vi "LSMcontroller_v56_from here for labview64bit.vi"() -> ()   [LabVIEW 2015] (continued)
                n2595 = call-poly <vilib>:"DAQmx Write.vi"("task/channels in"=w5605, "data"=w5596, "error in"=w5604) -> ("task out"=w5606:refnum<k21>, "error out"=w5607:errorcluster)  [unwired: 10 in, 1 out]
                n2596 = call <vilib>:"DAQmx Start Task.vi"("task/channels in"=w5606, "error in"=w5607) -> ("task out"=w5608:refnum<k21>, "error out"=w5609:errorcluster)  [unwired: 12 in]
                n2597 = call <vilib>:"DAQmx Stop Task.vi"("task/channels in"=w5608, "error in"=w5609) -> ("task out"=w5610:refnum<k21>, "error out"=w5611:errorcluster)  [unwired: 12 in]
                n2598 = call <vilib>:"DAQmx Clear Task.vi"("task in"=w5610, "error in"=w5611) -> ()  [unwired: 13 in, 1 out]
              }
            }
          }
          event "sealtest": Value Change {
            n2599 = event-data() -> ()  [unwired: 1 in, 6 out]
            n2600 = case shown="True" "sealtest" {
              frame False {
              }
              frame True {
                n2601 = stacked-sequence {
                  seq-local: [w5613 _ _ _ _ _] -> [_ w5646 _ w5698 _ _]
                  frame #0 {
                    n2602 = stacked-sequence {
                      tunnel: [_ w5625 _] -> w5613
                      frame #0 {
                        n2603 = call "2pparameters.vi"("command"="get") -> ("params out"=w5618:T12)  [unwired: 1 in]
                        n2604 = Unbundle By Name(w5618) -> ("autoshutter"=w5619:bool)
                        n2605 = local read "OCchecked?"() -> (w5616:bool)
                        n2606 = call "sealtestwfparams.vi"("command"="set") -> ()  [unwired: 6 in, 1 out]
                        n2607 = case shown="False" w5616 {
                          frame False {
                            n2608 = One Button Dialog(message="Is the OC gain correct?", button name ("OK")="ok") -> (true=w5620:bool)
                            n2609 = local write "OCchecked?"(w5620) -> ()
                          }
                          frame True {
                          }
                        }
                        n2610 = case shown="True" w5619 {
                          frame False {
                          }
                          frame True {
                            n2611 = call "shuttercontrol.vi"("command"="close") -> ()  [unwired: 1 in, 1 out]
                          }
                        }
                        n2612 = call "allAI-temp.vi"("command"=enum16{"get", "set", "clear", "append"}."clear") -> ()  [unwired: 3 in, 2 out]
                      }
                      frame #1 {
                        n2613 = call "sealtestwfparams.vi"("command"="get") -> ("Params out"=w5631:T25)  [unwired: 6 in]
                        n2614 = Unbundle By Name(w5631) -> ("AO parameters"=w5629:T1)
                        "AO parameters 2" <- w5629
                        n2615 = Index Array(array=w5629, index=0) -> (element=w5628:T26)
                        n2616 = call "generateRampedSquareWave_fromAOparameters.vi"("AO params"=w5628) -> ("Waveform"=w5624:waveform(dbl), "wflength"=w5625:i32)
                        "Waveform Graph" <- w5624
                        "wflength" <- w5625
                        n2617 = Build Array(w5624) -> (w5627:waveform(dbl)[])
                        n2618 = call "waveformssealtestbuffer.vi"("AO wf in"=w5627, "command"="set") -> ()  [unwired: 1 out]
                      }
                      frame #2 {
                        n2619 = local read "Vholding (mV)"() -> (w5634:sgl)
                        n2620 = local read "Current Clamp"() -> (w5640:bool)
                        n2621 = local read "Voltage Clamp"() -> (w5639:bool)
                        n2622 = local read "OCgain"() -> (w5635:sgl)
                        n2623 = local read "CC_ICgain"() -> (w5638:dbl)
                        n2624 = local read "holdon"() -> (w5633:bool)
                        n2625 = call "patchparameters.vi"("command"="get") -> ("Params out"=w5642:T15)  [unwired: 1 in]
                        n2626 = Bundle By Name(cluster=w5642, "VC"=w5639, "CC"=w5640, "CC_icg (pA/mv)"=w5638, "VC_icg (mV/mV)"=10.0, "OCG (mV/pA)"=w5635, "OVG (mV/mV)"=0.1, "Vhold (mV)"=w5634, "holdon"=w5633) -> (w5641:T15)
                        n2627 = call "patchparameters.vi"("Params in"=w5641, "command"="set") -> ()  [unwired: 1 out]
                      }
                    }
                  }
                  frame #1 {
                    w5645 = 2
                    n2628 = call "patchparameters.vi"("command"="get") -> ("Params out"=w5653:T15)  [unwired: 1 in]
                    n2629 = Unbundle By Name(w5653) -> ("holdon"=w5652:bool, "Vhold (mV)"=w5651:sgl, "CC_icg (pA/mv)"=w5659:sgl, "CC"=w5657:bool, "VC_icg (mV/mV)"=w5658:sgl)
                    n2630 = Select(t=w5659, s=w5657, f=w5658) -> (s? t:f=w5660:sgl)
                    n2631 = To Single Precision Float(number=0.001 ("y")) -> (single precision float=w5661:sgl)
                    n2632 = Compound Arithmetic op=MULTIPLY(w5651, w5660, w5661) -> (w5655:sgl)
                    n2633 = case shown="False" w5652 {
                      tunnel: w5655 -> [_ w5673]
                      tunnel: [0.0 w5673] -> w5648
                      frame False {
                      }
                      frame True {
                      }
                    }
                    n2634 = Greater Than 0?(x=w5645) -> (x > 0?=w5647:bool)
                    n2635 = case shown="True" w5647 {
                      tunnel: w5646 -> [_ w5662]
                      tunnel: w5645 -> [_ w5665]
                      frame False {
                      }
                      frame True {
                        n2636 = Initialize Array(sgl 0.0 ("element"), w5665, w5662) -> (w5663:sgl[][])
                        n2637 = call "allAI-temp.vi"("array in"=w5663, "command"=enum16{"get", "set", "clear", "append"}."set") -> ()  [unwired: 2 in, 2 out]
                      }
                    }
                    n2638 = flat-sequence {
                      tunnel: w5646 -> [w5669]
                      tunnel: w5646 -> [w5668]
                      tunnel: [w5668] -> w5650
                      tunnel: [w5667] -> w5649
                      tunnel: w5648 -> [w5667]
                      tunnel: w5650 -> [w5671]
                      tunnel: w5649 -> [w5670]
                      frame #0 {
                        n2639 = call "prepAI_sealtest.vi"("samples per channel"=w5669) -> ()  [unwired: 2 in]
                      }
                      frame #1 {
                        n2640 = call "prepAO_sealtest.vi"("Vhold"=w5670, "samples per channel"=w5671) -> ()  [unwired: 1 in]
                      }
                    }
                  }
                  frame #2 {
                    n2641 = stacked-sequence {
                      frame #0 {
                        n2642 = call "tempconfigAO.vi"("command"="get") -> ("Temp Config out"=w5677:T27)  [unwired: 1 in]
                        n2643 = Unbundle By Name(w5677) -> ("AO"=w5678:refnum<k21>[], "E_AO"=w5679:errorcluster[])
                        n2644 = for {
                          tunnel: w5678 -> [w5687] mode=indexing
                          tunnel: w5679 -> [w5686] mode=indexing
                          tunnel: [w5685] -> w5681 mode=indexing
                          tunnel: [w5684] -> w5682 mode=indexing
                          n2645 = call <vilib>:"DAQmx Start Task.vi"("task/channels in"=w5687, "error in"=w5686) -> ("task out"=w5685:refnum<k21>, "error out"=w5684:errorcluster)  [unwired: 12 in]
                        }
                        n2646 = call "tempconfigAO.vi"("command"="get") -> ("Temp Config out"=w5680:T27)  [unwired: 1 in]
                        n2647 = Bundle By Name(cluster=w5680, "AO"=w5681, "E_AO"=w5682) -> (w5683:T27)
                        n2648 = call "tempconfigAO.vi"("Temp Config in"=w5683, "command"="set") -> ()  [unwired: 1 out]
                      }
                      frame #1 {
                        n2649 = call "tempconfigAI.vi"("command"="get") -> ("Temp Config out"=w5689:T28)  [unwired: 1 in]
                        n2650 = Unbundle By Name(w5689) -> ("AI"=w5694:refnum<k21>, "E_AI"=w5695:errorcluster)
                        n2651 = call <vilib>:"DAQmx Start Task.vi"("task/channels in"=w5694, "error in"=w5695) -> ("task out"=w5696:refnum<k21>, "error out"=w5697:errorcluster)  [unwired: 12 in]
                        n2652 = call "tempconfigAI.vi"("command"="get") -> ("Temp Config out"=w5691:T28)  [unwired: 1 in]
                        n2653 = Bundle By Name(cluster=w5691, "AI"=w5696, "E_AI"=w5697) -> (w5693:T28)
                        n2654 = call "tempconfigAI.vi"("Temp Config in"=w5693, "command"="set") -> ()  [unwired: 1 out]
                      }
                    }
                  }
                  frame #3 {
                    n2655 = while {
                      tunnel: w5698 -> [w5699]
                      stop <- w5700 stop-if-true
                      n2656 = local read "sealtest"() -> (w5703:bool)
                      n2657 = Not(x=w5703) -> (.not. x?=w5702:bool)
                      n2658 = case shown="False" w5702 {
                        tunnel: w5699 -> [w5704 _]
                        frame False {
                          n2659 = stacked-sequence {
                            seq-local: [_ _ _ w5743 _ _] -> [_ _ _ _ w5799 _]
                            seq-local: [w5705 _ _ _ _ _] -> [_ w5714 _ w5736 w5784 w5819]
                            tunnel: w5704 -> [_ _ w5722 _ w5783 _]
                            frame #0 {
                              n2660 = call "patchparameters.vi"("command"="get") -> ("Params out"=w5712:T15)  [unwired: 1 in]
                              n2661 = local read "Vholding (mV)"() -> (w5709:sgl)
                              n2662 = Unbundle By Name(w5712) -> ("Vhold (mV)"=w5708:sgl, "holdon"=w5711:bool)
                              n2663 = local read "holdon"() -> (w5710:bool)
                              n2664 = Not Equal?(x=w5709, y=w5708) -> (x != y?=w5707:bool)
                              n2665 = Not Equal?(x=w5711, y=w5710) -> (x != y?=w5706:bool)
                              n2666 = Or(x=w5707, y=w5706) -> (x .or. y?=w5705:bool)
                            }
                            frame #1 {
                              n2667 = case shown="True" w5714 {
                                frame False {
                                }
                                frame True {
                                n2668 = local read "Vholding (mV)"() -> (w5717:sgl)
                                n2669 = local read "holdon"() -> (w5715:bool)
                                n2670 = call "patchparameters.vi"("command"="get") -> ("Params out"=w5718:T15)  [unwired: 1 in]
                                n2671 = Bundle By Name(cluster=w5718, "Vhold (mV)"=w5717, "holdon"=w5715) -> (w5716:T15)
                                n2672 = call "patchparameters.vi"("Params in"=w5716, "command"="set") -> ()  [unwired: 1 out]
                                }
                              }
                            }
                            frame #2 {
                              n2673 = call "tempconfigAI.vi"("command"="get") -> ("Temp Config out"=w5732:T28)  [unwired: 1 in]
                              n2674 = Unbundle By Name(w5732) -> ("AI"=w5731:refnum<k21>, "E_AI"=w5730:errorcluster)
                              n2675 = call-poly <vilib>:"DAQmx Read.vi"("task/channels in"=w5731, "number of samples per channel"=w5722, "timeout"=10.0, "error in"=w5730) -> ("task out"=w5726:refnum<k21>, "data"=w5723:i16[][], "error out"=w5735:errorcluster)  [unwired: 9 in]
                              n2676 = call "tempconfigAI.vi"("command"="get") -> ("Temp Config out"=w5727:T28)  [unwired: 1 in]
                              n2677 = Bundle By Name(cluster=w5727, "AI"=w5726, "E_AI"=w5735) -> (w5734:T28)
                              n2678 = To Single Precision Float(number=w5723) -> (single precision float=w5725:sgl[][])
                              n2679 = call "tempconfigAI.vi"("Temp Config in"=w5734, "command"="set") -> ()  [unwired: 1 out]
                              n2680 = call "allAI-temp.vi"("array in"=w5725, "command"=enum16{"get", "set", "clear", "append"}."set") -> ()  [unwired: 2 in, 2 out]
                            }
                            frame #3 {
                              n2681 = case shown="True" w5736 {
                                frame False {
                                }
                                frame True {
                                n2682 = call "tempconfigAO.vi"("command"="get") -> ("Temp Config out"=w5776:T27)  [unwired: 1 in]
                                n2683 = Unbundle By Name(w5776) -> ("AO"=w5775:refnum<k21>[], "E_AO"=w5774:errorcluster[])
                                n2684 = call "tempconfigAI.vi"("command"="get") -> ("Temp Config out"=w5763:T28)  [unwired: 1 in]
                                n2685 = Unbundle By Name(w5763) -> ("AI"=w5764:refnum<k21>, "E_AI"=w5765:errorcluster)
                                n2686 = for {
                                tunnel: w5775 -> [w5780] mode=indexing
                                tunnel: w5774 -> [w5779] mode=indexing
                                tunnel: [w5778] -> w5770 mode=indexing
                                n2687 = call <vilib>:"DAQmx Stop Task.vi"("task/channels in"=w5780, "error in"=w5779) -> ("task out"=w5781:refnum<k21>, "error out"=w5782:errorcluster)  [unwired: 12 in]
                                n2688 = call <vilib>:"DAQmx Clear Task.vi"("task in"=w5781, "error in"=w5782) -> ("error out"=w5778:errorcluster)  [unwired: 13 in]
                                }
                                n2689 = call <vilib>:"DAQmx Stop Task.vi"("task/channels in"=w5764, "error in"=w5765) -> ("task out"=w5761:refnum<k21>, "error out"=w5760:errorcluster)  [unwired: 12 in]
                                n2690 = call <vilib>:"DAQmx Clear Task.vi"("task in"=w5761, "error in"=w5760) -> ("error out"=w5759:errorcluster)  [unwired: 13 in]
                                n2691 = call "tempconfigAO.vi"("command"="get") -> ("Temp Config out"=w5771:T27)  [unwired: 1 in]
                                n2692 = Bundle By Name(cluster=w5771, "E_AO"=w5770) -> (w5769:T27)
                                n2693 = call "tempconfigAI.vi"("command"="get") -> ("Temp Config out"=w5767:T28)  [unwired: 1 in]
                                n2694 = Bundle By Name(cluster=w5767, "E_AI"=w5759) -> (w5758:T28)
                                n2695 = call "tempconfigAO.vi"("Temp Config in"=w5769, "command"="set") -> ()  [unwired: 1 out]
                                n2696 = call "tempconfigAI.vi"("Temp Config in"=w5758, "command"="set") -> ()  [unwired: 1 out]
                                }
                              }
                              n2697 = call "allAI-temp.vi"("command"=enum16{"get", "set", "clear", "append"}."get") -> ("array out"=w5740:sgl[][])  [unwired: 3 in, 1 out]
                              n2698 = call "tempconfigAI.vi"("command"="get") -> ("Temp Config out"=w5753:T28)  [unwired: 1 in]
                              n2699 = call "tempconfigAI.vi"("command"="get") -> ("Temp Config out"=w5755:T28)  [unwired: 1 in]
                              n2700 = Unbundle By Name(w5753) -> ("header"=w5751:dbl[])
                              n2701 = Unbundle By Name(w5755) -> ("header"=w5757:dbl[])
                              n2702 = Index Array(array=w5740, index (row) #1=0 ("index (row)"), index (row) #2=1 ("index (row)")) -> (element #1=w5738:sgl[], element #2=w5737:sgl[])  [unwired: 2 in]
                              n2703 = local read "OCgain"() -> (w5745:sgl)
                              n2704 = call "Unscaledtoscaled.vi"("Unscaled Data"=w5738, "Header Information"=w5751) -> ("Array"=w5750:sgl[])  [unwired: 1 in]
                              n2705 = call "Unscaledtoscaled.vi"("Unscaled Data"=w5737, "Header Information"=w5757) -> ("Array"=w5754:sgl[])  [unwired: 1 in]
                              n2706 = Multiply(x=w5750, y=0.1) -> (x*y=w5747:dbl[])
                              n2707 = Divide(x=w5754, y=w5745) -> (x/y=w5746:sgl[])
                              n2708 = Build Array(w5747, w5746) -> (w5749:dbl[][])
                              n2709 = Multiply(x=w5749, y=1000.0) -> (x*y=w5743:dbl[][])
                              "Patch readout" <- w5743
                            }
                            frame #4 {
                              n2710 = case shown="True" w5784 {
                                tunnel: w5783 -> [_ w5800]
                                frame False {
                                }
                                frame True {
                                n2711 = call "patchparameters.vi"("command"="get") -> ("Params out"=w5804:T15)  [unwired: 1 in]
                                n2712 = Unbundle By Name(w5804) -> ("holdon"=w5803:bool, "Vhold (mV)"=w5802:sgl, "CC_icg (pA/mv)"=w5810:sgl, "CC"=w5808:bool, "VC_icg (mV/mV)"=w5809:sgl)
                                n2713 = Select(t=w5810, s=w5808, f=w5809) -> (s? t:f=w5811:sgl)
                                n2714 = To Single Precision Float(number=0.001 ("y")) -> (single precision float=w5812:sgl)
                                n2715 = Compound Arithmetic op=MULTIPLY(w5802, w5811, w5812) -> (w5806:sgl)
                                n2716 = case shown="False" w5803 {
                                tunnel: w5806 -> [_ w5817]
                                tunnel: [0.0 w5817] -> w5801
                                frame False {
                                }
                                frame True {
                                }
                                }
                                n2717 = flat-sequence {
                                tunnel: w5800 -> [w5813]
                                tunnel: w5801 -> [w5815]
                                tunnel: w5800 -> [w5814]
                                frame #0 {
                                n2718 = call "prepAI_sealtest.vi"("samples per channel"=w5813) -> ()  [unwired: 2 in]
                                }
                                frame #1 {
                                n2719 = call "prepAO_sealtest.vi"("Vhold"=w5815, "samples per channel"=w5814) -> ()  [unwired: 1 in]
                                }
                                }
                                }
                              }
                              n2720 = call "sealtestwfparams.vi"("command"="get") -> ("Params out"=w5789:T25)  [unwired: 6 in]
                              n2721 = Unbundle By Name(w5789) -> ("AO parameters"=w5790:T1)
                              n2722 = Index Array(array=w5790, index=0) -> (element=w5792:T26)
                              n2723 = Unbundle By Name(w5792) -> ("Cycles"=w5787:dbl, "Start amplitude (V)"=w5786:dbl, "Sampling frequency (Hz)"=w5785:dbl)
                              n2724 = local read "fitpoints"() -> (w5794:dbl)
                              n2725 = script code="V=data(:,2);\nI=data(:,1);\ntres=mean(V);\nspc=(nsamp./ncyc);\nV=V(spc+1:end-spc);\nI=I(spc+1:end-spc);\ndV=mean(V(V>tres))-mean(V(V<tres))\nIcyc=reshape(I,[spc ncyc-2]);\nIcyc=Icyc';\nIcyc=mean(Icyc,1);\ndIss=mean(Icyc(floor(spc*0.15):floor(spc/2)-2))-mean(Icyc(spc*0.65:spc-2))\nRm=dV*1e3/dIss;\n[maxi,ind]=max(Icyc);\nIfit=Icyc(ind+1:ind+1+points-1)-0.5*(mean(Icyc(floor(spc*0.15):floor(spc/2)-2))+mean(Icyc(spc*0.65:spc-2)))\nt=(3:points-1+3)./srate*1000;\nt=t';\nIfit=Ifit';\nc=fit(t,Ifit, 'exp1');\ncoeffs=coeffvalues(c);\nIa=coeffs(1);\nRa=dV*1e3./Ia/2;\ntau=-1./coeffs(2);\ncap=tau/Ra*1000;"("data"=w5799, "nsamp"=w5783, "ncyc"=w5787, "maxV"=w5786, "points"=w5794, "srate"=w5785) -> ("Icyc"=w5798:dbl[], "Rm"=w5796:dbl, "Ra"=w5795:dbl, "cap"=w5793:dbl)  [unwired: 1 in, 1 out]
                              n2726 = local read "set as Rp?"() -> (w5797:bool)
                              n2727 = local write "Rmembrane (MOhm)"(w5796) -> ()
                              n2728 = case shown="True" w5797 {
                                tunnel: w5796 -> [_ w5818]
                                frame False {
                                }
                                frame True {
                                n2729 = local write "Rpipette (MOhm)"(w5818) -> ()
                                }
                              }
                              n2730 = local write "Cmembrane"(w5793) -> ()
                              n2731 = local write "Racces (MOhm)"(w5795) -> ()
                              n2732 = local write "Ifit"(w5798) -> ()
                            }
                            frame #5 {
                              n2733 = local read "set as Rp?"() -> (w5820:bool)
                              n2734 = case shown="True" w5819 {
                                frame False {
                                }
                                frame True {
                                n2735 = call "tempconfigAO.vi"("command"="get") -> ("Temp Config out"=w5827:T27)  [unwired: 1 in]
                                n2736 = Unbundle By Name(w5827) -> ("AO"=w5826:refnum<k21>[], "E_AO"=w5825:errorcluster[])
                                n2737 = call "tempconfigAI.vi"("command"="get") -> ("Temp Config out"=w5832:T28)  [unwired: 1 in]
                                n2738 = Unbundle By Name(w5832) -> ("AI"=w5837:refnum<k21>, "E_AI"=w5838:errorcluster)
                                n2739 = for {
                                tunnel: w5826 -> [w5844] mode=indexing
                                tunnel: w5825 -> [w5843] mode=indexing
                                tunnel: [w5842] -> w5823 mode=indexing
                                tunnel: [w5841] -> w5822 mode=indexing
                                n2740 = call <vilib>:"DAQmx Start Task.vi"("task/channels in"=w5844, "error in"=w5843) -> ("task out"=w5842:refnum<k21>, "error out"=w5841:errorcluster)  [unwired: 12 in]
                                }
                                n2741 = call <vilib>:"DAQmx Start Task.vi"("task/channels in"=w5837, "error in"=w5838) -> ("task out"=w5839:refnum<k21>, "error out"=w5840:errorcluster)  [unwired: 12 in]
                                n2742 = call "tempconfigAO.vi"("command"="get") -> ("Temp Config out"=w5824:T27)  [unwired: 1 in]
                                n2743 = call "tempconfigAI.vi"("command"="get") -> ("Temp Config out"=w5834:T28)  [unwired: 1 in]
                                n2744 = Bundle By Name(cluster=w5824, "AO"=w5823, "E_AO"=w5822) -> (w5821:T27)
                                n2745 = Bundle By Name(cluster=w5834, "AI"=w5839, "E_AI"=w5840) -> (w5836:T28)
                                n2746 = call "tempconfigAI.vi"("Temp Config in"=w5836, "command"="set") -> ()  [unwired: 1 out]
                                n2747 = call "tempconfigAO.vi"("Temp Config in"=w5821, "command"="set") -> ()  [unwired: 1 out]
                                }
                              }
                              n2748 = case shown="True" w5820 {
                                frame False {
                                }
                                frame True {
                                n2749 = local write "set as Rp?"(FALSE ("set as Rp?")) -> ()
                                }
                              }
                            }
                          }
                        }
                        frame True {
                        }
                      }
                      n2750 = local read "sealtest"() -> (w5701:bool)
                      n2751 = Not(x=w5701) -> (.not. x?=w5700:bool)
                    }
                  }
                  frame #4 {
                    n2752 = call "tempconfigAO.vi"("command"="get") -> ("Temp Config out"=w5871:T27)  [unwired: 1 in]
                    n2753 = Unbundle By Name(w5871) -> ("AO"=w5870:refnum<k21>[], "E_AO"=w5869:errorcluster[])
                    n2754 = call "configuration.vi"("command"="get") -> ("config out"=w5852:T13)  [unwired: 2 in, 1 out]
                    n2755 = call "tempconfigAI.vi"("command"="get") -> ("Temp Config out"=w5858:T28)  [unwired: 1 in]
                    n2756 = Unbundle By Name(w5852) -> ("Device 1 sampleclock out"=w5849:tag, "Device 1 Starttrigger out"=w5848:tag)
                    n2757 = Unbundle By Name(w5858) -> ("AI"=w5859:refnum<k21>, "E_AI"=w5860:errorcluster)
                    n2758 = for {
                      tunnel: w5870 -> [w5875] mode=indexing
                      tunnel: w5869 -> [w5874] mode=indexing
                      tunnel: [w5873] -> w5865 mode=indexing
                      n2759 = call <vilib>:"DAQmx Stop Task.vi"("task/channels in"=w5875, "error in"=w5874) -> ("task out"=w5876:refnum<k21>, "error out"=w5877:errorcluster)  [unwired: 12 in]
                      n2760 = call <vilib>:"DAQmx Clear Task.vi"("task in"=w5876, "error in"=w5877) -> ("error out"=w5873:errorcluster)  [unwired: 13 in]
                    }
                    n2761 = call <vilib>:"DAQmx Stop Task.vi"("task/channels in"=w5859, "error in"=w5860) -> ("task out"=w5856:refnum<k21>, "error out"=w5855:errorcluster)  [unwired: 12 in]
                    n2762 = call <vilib>:"DAQmx Disconnect Terminals.vi"("source terminal"=tag "/Dev1/ai/SampleClock", "destination terminal"=w5849) -> ("error out"=w5846:errorcluster)  [unwired: 13 in]
                    n2763 = call <vilib>:"DAQmx Clear Task.vi"("task in"=w5856, "error in"=w5855) -> ("error out"=w5854:errorcluster)  [unwired: 13 in]
                    n2764 = call "tempconfigAO.vi"("command"="get") -> ("Temp Config out"=w5866:T27)  [unwired: 1 in]
                    n2765 = Bundle By Name(cluster=w5866, "E_AO"=w5865) -> (w5864:T27)
                    n2766 = call "tempconfigAI.vi"("command"="get") -> ("Temp Config out"=w5862:T28)  [unwired: 1 in]
                    n2767 = Bundle By Name(cluster=w5862, "E_AI"=w5854) -> (w5853:T28)
                    n2768 = call "tempconfigAO.vi"("Temp Config in"=w5864, "command"="set") -> ()  [unwired: 1 out]
                    n2769 = call <vilib>:"DAQmx Disconnect Terminals.vi"("source terminal"=tag "/Dev1/ai/StartTrigger", "destination terminal"=w5848, "error in"=w5846) -> ()  [unwired: 12 in, 1 out]
                    n2770 = call "tempconfigAI.vi"("Temp Config in"=w5853, "command"="set") -> ()  [unwired: 1 out]
                  }
                  frame #5 {
                    w5880 = T23 4 items=["no dialog", "OK message", "continue or stop message", "OK message + warnings", "continue/stop + warnings"] ("type of dialog (OK msg:1)")
                    n2771 = call "displayerrors.vi"() -> ("error IO"=w5879:errorcluster)
                    n2772 = call "zeropatch.vi"() -> ()  [unwired: 12 in]
                    n2773 = call <vilib>:"Simple Error Handler.vi"("type of dialog (OK msg:1)"=w5880, "error in (no error)"=w5879) -> ("error out"=w5878:errorcluster)  [unwired: 3 in, 4 out]
                    n2774 = call <vilib>:"Clear Errors.vi"("error in (no error)"=w5878) -> ()  [unwired: 5 in, 2 out]
                  }
                }
              }
            }
          }
          event "Current Clamp": Value Change {
            n2775 = event-data() -> ()  [unwired: 1 in, 6 out]
            n2776 = local read "Current Clamp"() -> (w5885:bool)
            n2777 = property on="Vholding (mV)" class="DigNum (strict)"("Caption.Text"="Ihold (pA)") -> ()  [unwired: 2 in, 2 out]
            n2778 = Not(x=w5885) -> (.not. x?=w5884:bool)
            n2779 = property on="Voltage Clamp" class="Bool (strict)"("Value"=w5884) -> ()  [unwired: 2 in, 2 out]
            n2780 = One Button Dialog(message="Have you switched the HEKA to CC and changed the external input cable?", button name ("OK")="Ok") -> ()  [unwired: 1 out]
          }
          event "Voltage Clamp": Value Change {
            n2781 = event-data() -> ()  [unwired: 1 in, 6 out]
            n2782 = local read "Voltage Clamp"() -> (w5890:bool)
            n2783 = Not(x=w5890) -> (.not. x?=w5889:bool)
            n2784 = property on="Current Clamp" class="Bool (strict)"("Value"=w5889) -> ()  [unwired: 2 in, 2 out]
            n2785 = One Button Dialog(message="Have you switched the HEKA to VC and changed the external input cable?", button name ("OK")="Ok") -> ()  [unwired: 1 out]
            n2786 = property on="Vholding (mV)" class="DigNum (strict)"("Caption.Text"="Vhold (mV)") -> ()  [unwired: 2 in, 2 out]
          }
          event "OCgain": Value Change {
            n2787 = event-data() -> ()  [unwired: 1 in, 6 out]
            n2788 = local read "OCgain"() -> (w5893:sgl)
            n2789 = Less?(x=w5893, y=0.3) -> (x < y?=w5891:bool)
            n2790 = case shown="True" w5891 {
              frame False {
                w5894 = 10.0 items=["0.1"=10.0, "10"=0.1] ("CC_ICgain")
                n2791 = local write "CC_ICgain"(w5894) -> ()
              }
              frame True {
                w5895 = 0.1 items=["0.1"=10.0, "10"=0.1] ("CC_ICgain")
                n2792 = local write "CC_ICgain"(w5895) -> ()
              }
            }
          }
          event "holdon": Value Change {
            n2793 = event-data() -> ()  [unwired: 1 in, 6 out]
            n2794 = stacked-sequence {
              frame #0 {
                n2795 = local read "Vholding (mV)"() -> (w5899:sgl)
                n2796 = local read "holdon"() -> (w5896:bool)
                n2797 = call "patchparameters.vi"("command"="get") -> ("Params out"=w5900:T15)  [unwired: 1 in]
                n2798 = Bundle By Name(cluster=w5900, "Vhold (mV)"=w5899, "holdon"=w5896) -> (w5897:T15)
                n2799 = call "patchparameters.vi"("Params in"=w5897, "command"="set") -> ()  [unwired: 1 out]
              }
              frame #1 {
                n2800 = call "zeropatch.vi"() -> ()  [unwired: 12 in]
              }
            }
          }
          event "Vholding (mV)": Value Change {
            n2801 = event-data() -> ()  [unwired: 1 in, 6 out]
            n2802 = local read "holdon"() -> (w5902:bool)
            n2803 = case shown="True" w5902 {
              frame False {
              }
              frame True {
                n2804 = stacked-sequence {
                  frame #0 {
                    n2805 = local read "Vholding (mV)"() -> (w5905:sgl)
                    n2806 = local read "holdon"() -> (w5906:bool)
                    n2807 = call "patchparameters.vi"("command"="get") -> ("Params out"=w5907:T15)  [unwired: 1 in]
                    n2808 = Bundle By Name(cluster=w5907, "Vhold (mV)"=w5905, "holdon"=w5906) -> (w5903:T15)
                    n2809 = call "patchparameters.vi"("Params in"=w5903, "command"="set") -> ()  [unwired: 1 out]
                  }
                  frame #1 {
                    n2810 = call "zeropatch.vi"() -> ()  [unwired: 12 in]
                  }
                }
              }
            }
          }
          event "readpatch": Value Change {
            n2811 = event-data() -> ("NewVal"=w5909:bool)  [unwired: 1 in, 5 out]
            n2812 = case shown="True" w5909 {
              frame False {
              }
              frame True {
                n2813 = stacked-sequence {
                  frame #0 {
                    n2814 = stacked-sequence {
                      frame #0 {
                        n2815 = call "2pparameters.vi"("command"="get") -> ("params out"=w5911:T12)  [unwired: 1 in]
                        n2816 = Unbundle By Name(w5911) -> ("autoshutter"=w5912:bool)
                        n2817 = case shown="True" w5912 {
                          frame False {
                          }
                          frame True {
                            n2818 = call "shuttercontrol.vi"("command"="close") -> ()  [unwired: 1 in, 1 out]
                          }
                        }
                      }
                      frame #1 {
                        n2819 = local read "Voltage Clamp"() -> (w5919:bool)
                        n2820 = local read "Current Clamp"() -> (w5920:bool)
                        n2821 = local read "Vholding (mV)"() -> (w5914:sgl)
                        n2822 = local read "CC_ICgain"() -> (w5918:dbl)
                        n2823 = local read "OCgain"() -> (w5915:sgl)
                        n2824 = call "patchparameters.vi"("command"="get") -> ("Params out"=w5922:T15)  [unwired: 1 in]
                        n2825 = Bundle By Name(cluster=w5922, "VC"=w5919, "CC"=w5920, "CC_icg (pA/mv)"=w5918, "VC_icg (mV/mV)"=10.0, "OCG (mV/pA)"=w5915, "OVG (mV/mV)"=0.1, "Vhold (mV)"=w5914) -> (w5921:T15)
                        n2826 = call "patchparameters.vi"("Params in"=w5921, "command"="set") -> ()  [unwired: 1 out]
                      }
                      frame #2 {
                        w5933 = 10123 items=["Finite Samples"=10178, "Continuous Samples"=10123, "Hardware Timed Single Point"=12522] ("sample mode")
                        n2827 = call "configuration.vi"("command"="get") -> ("config out"=w5928:T13)  [unwired: 2 in, 1 out]
                        n2828 = Unbundle By Name(w5928) -> ("Vp"=w5927:i32, "Ip"=w5926:i32)
                        n2829 = call "2pparameters.vi"("command"="get") -> ("params out"=w5936:T12)  [unwired: 1 in]
                        n2830 = Build Array(w5927, w5926) -> (w5925:i32[])
                        n2831 = Bundle By Name(cluster=w5936, "srate"=10000.0, "refreshbuffer"=500, "timeout"=10.0, "sample mode"=w5933, "aAI"=w5925) -> (w5934:T12)
                        n2832 = call "2pparameters.vi"("Params in"=w5934, "command"="set") -> ()  [unwired: 1 out]
                      }
                    }
                  }
                  frame #1 {
                    n2833 = while {
                      stop <- w5938 stop-if-true
                      n2834 = local read "readpatch"() -> (w5940:bool)
                      n2835 = case shown="True" w5940 {
                        frame False {
                        }
                        frame True {
                          n2836 = stacked-sequence {
                            frame #0 {
                              n2837 = local read "Vholding (mV)"() -> (w5943:sgl)
                              n2838 = local read "holdon"() -> (w5941:bool)
                              n2839 = call "patchparameters.vi"("command"="get") -> ("Params out"=w5944:T15)  [unwired: 1 in]
                              n2840 = Bundle By Name(cluster=w5944, "Vhold (mV)"=w5943, "holdon"=w5941) -> (w5942:T15)
                              n2841 = call "patchparameters.vi"("Params in"=w5942, "command"="set") -> ()  [unwired: 1 out]
                            }
                            frame #1 {
                              n2842 = call "zeropatch.vi"() -> ()  [unwired: 12 in]
                            }
                            frame #2 {
                              n2843 = call "prepAI_ttv2.vi"() -> ()  [unwired: 2 in, 1 out]
                            }
                            frame #3 {
                              n2844 = call "runAI_tt.vi"() -> ()  [unwired: 12 in]
                            }
                            frame #4 {
                              n2845 = call "collectAI_tt_V2.vi"() -> ()  [unwired: 4 in]
                            }
                            frame #5 {
                              n2846 = call "stoperaseAI_tt.vi"() -> ()  [unwired: 12 in]
                            }
                            frame #6 {
                              n2847 = call "tempconfigAI.vi"("command"="get") -> ("Temp Config out"=w5962:T28)  [unwired: 1 in]
                              n2848 = Unbundle By Name(w5962) -> ("header"=w5952:dbl[])
                              n2849 = call "allAI-temp.vi"("command"=enum16{"get", "set", "clear", "append"}."get") -> ("array out"=w5953:sgl[][])  [unwired: 3 in, 1 out]
                              n2850 = call "Unscaledtoscaled2D.vi"("Unscaled Data"=w5953, "Header Information"=w5952) -> ("Array"=w5951:sgl[][])  [unwired: 1 in]
                              n2851 = local read "OCgain"() -> (w5963:sgl)
                              n2852 = Index Array(array=w5951, index (row) #1=0 ("index (row)"), index (row) #2=1 ("index (row)")) -> (element #1=w5948:sgl[], element #2=w5947:sgl[])  [unwired: 2 in]
                              n2853 = Divide(x=w5948, y=w5963) -> (x/y=w5957:sgl[])
                              n2854 = Multiply(x=w5947, y=sgl 0.1) -> (x*y=w5956:sgl[])
                              n2855 = Build Array(w5957, w5956) -> (w5960:sgl[][])
                              n2856 = Multiply(x=w5960, y=sgl 1000.0) -> (x*y=w5955:sgl[][])
                              n2857 = local write "Patch readout"(w5955) -> ()
                            }
                          }
                        }
                      }
                      n2858 = local read "readpatch"() -> (w5939:bool)
                      n2859 = Not(x=w5939) -> (.not. x?=w5938:bool)
                    }
                  }
                  frame #2 {
                    w5966 = T23 4 items=["no dialog", "OK message", "continue or stop message", "OK message + warnings", "continue/stop + warnings"] ("type of dialog (OK msg:1)")
                    n2860 = call "displayerrors.vi"() -> ("error IO"=w5965:errorcluster)
                    n2861 = call <vilib>:"Simple Error Handler.vi"("type of dialog (OK msg:1)"=w5966, "error in (no error)"=w5965) -> ("error out"=w5964:errorcluster)  [unwired: 3 in, 4 out]
                    n2862 = call <vilib>:"Clear Errors.vi"("error in (no error)"=w5964) -> ()  [unwired: 5 in, 2 out]
                  }
                  frame #3 {
                    n2863 = call "zeropatch.vi"() -> ()  [unwired: 12 in]
                  }
                  frame #4 {
                    n2864 = disable-structure shown="Disabled" {
                      frame Disabled {
                        n2865 = local read item#-1() -> (w5972)
                        n2866 = local read item#-1() -> (w5971)
                        n2867 = local read item#-1() -> (w5968)
                        n2868 = local read item#-1() -> (w5970)
                        n2869 = local read item#-1() -> (w5969)
                        n2870 = local read item#-1() -> (w5967)
                        n2871 = call "waveformparamsv2.vi"("command"="get") -> ("Params out"=w5974:T24)  [unwired: 1 in]
                        n2872 = Bundle By Name(cluster=w5974, "patch"=w5972, "laserAO"=w5971, "shutter"=w5970, "488"=w5969, "532"=w5968, "640"=w5967) -> (w5973:T24)
                        n2873 = call "waveformparamsv2.vi"("Params in"=w5973, "command"="set") -> ()  [unwired: 1 out]
                      }
                      frame Enabled {
                      }
                    }
                  }
                  frame #5 {
                    n2874 = call "2pparameters.vi"("command"="get") -> ("params out"=w5978:T12)  [unwired: 1 in]
                    n2875 = Unbundle By Name(w5978) -> ("autoshutter"=w5979:bool)
                    n2876 = case shown="True" w5979 {
                      frame False {
                      }
                      frame True {
                        n2877 = call "shuttercontrol.vi"("command"="close") -> ()  [unwired: 1 in, 1 out]
                      }
                    }
                  }
                }
              }
            }
          }
          event "AI channels": Value Change {
            n2878 = event-data() -> ()  [unwired: 1 in, 6 out]
            n2879 = local read "CI channels"() -> (w5988:i32[])
            n2880 = local read "AI channels"() -> (w5989:i32[])
            n2881 = call "configuration.vi"("command"="get") -> ("config out"=w5982:T13)  [unwired: 2 in, 1 out]
            n2882 = Unbundle By Name(w5982) -> ("CI names"=w5983:string[], "AI names"=w5984:string[])
            n2883 = for {
              tunnel: w5988 -> [w5994] mode=indexing
              tunnel: w5983 -> [w5995]
              tunnel: [w5993] -> w5985 mode=indexing
              n2884 = Index Array(array=w5995, index=w5994) -> (element=w5993:string)
            }
            n2885 = for {
              tunnel: w5989 -> [w5991] mode=indexing
              tunnel: w5984 -> [w5992]
              tunnel: [w5990] -> w5986 mode=indexing
              n2886 = Index Array(array=w5992, index=w5991) -> (element=w5990:string)
            }
            n2887 = Build Array (concatenate)(w5985, w5986) -> (w5987:string[])
            n2888 = property on="image1list" class="Ring (strict)"("Strings []"=w5987) -> ()  [unwired: 2 in, 2 out]
            n2889 = property on="image2list" class="Ring (strict)"("Strings []"=w5987) -> ()  [unwired: 2 in, 2 out]
          }
          event "CI channels": Value Change {
            n2890 = event-data() -> ()  [unwired: 1 in, 6 out]
            n2891 = local read "CI channels"() -> (w6003:i32[])
            n2892 = local read "AI channels"() -> (w6004:i32[])
            n2893 = call "configuration.vi"("command"="get") -> ("config out"=w5997:T13)  [unwired: 2 in, 1 out]
            n2894 = Unbundle By Name(w5997) -> ("CI names"=w5998:string[], "AI names"=w5999:string[])
            n2895 = for {
              tunnel: w6003 -> [w6009] mode=indexing
              tunnel: w5998 -> [w6010]
              tunnel: [w6008] -> w6000 mode=indexing
              n2896 = Index Array(array=w6010, index=w6009) -> (element=w6008:string)
            }
            n2897 = for {
              tunnel: w6004 -> [w6006] mode=indexing
              tunnel: w5999 -> [w6007]
              tunnel: [w6005] -> w6001 mode=indexing
              n2898 = Index Array(array=w6007, index=w6006) -> (element=w6005:string)
            }
            n2899 = Build Array (concatenate)(w6000, w6001) -> (w6002:string[])
            n2900 = property on="image1list" class="Ring (strict)"("Strings []"=w6002) -> ()  [unwired: 2 in, 2 out]
            n2901 = property on="image2list" class="Ring (strict)"("Strings []"=w6002) -> ()  [unwired: 2 in, 2 out]
          }
          event "setdatdir": Value Change {
            n2902 = event-data() -> ()  [unwired: 1 in, 5 out]
            n2903 = case shown="True" "setdatdir" {
              frame False {
              }
              frame True {
                n2904 = stacked-sequence {
                  frame #0 {
                    n2905 = local read "data dir"() -> (w6012:path)
                    n2906 = call "File Dialog"("start path"=w6012, "prompt"="Please select data directory...") -> ("selected path"=w6014:path, "cancelled"=w6013:bool, "error out"=w6015:errorcluster)  [unwired: 10 in, 1 out]
                    n2907 = case shown="False" w6013 {
                      tunnel: w6014 -> [w6023 _]
                      tunnel: w6015 -> [w6020 w6026]
                      tunnel: [w6018 w6026] -> w6017
                      frame False {
                        n2908 = local write "data dir"(w6023) -> ()
                        n2909 = call "configuration.vi"("error in"=w6020, "command"="get") -> ("Error out"=w6019:errorcluster, "config out"=w6025:T13)  [unwired: 1 in]
                        n2910 = Bundle By Name(cluster=w6025, "master data dir"=w6023) -> (w6024:T13)
                        n2911 = call "configuration.vi"("error in"=w6019, "config in"=w6024, "command"="set") -> ("Error out"=w6018:errorcluster)  [unwired: 1 out]
                      }
                      frame True {
                      }
                    }
                    n2912 = local write "status"(w6017) -> ()
                  }
                  frame #1 {
                    n2913 = property on="setdatdir" class="Bool (strict)"("Value"=FALSE ("setdatdir")) -> ()  [unwired: 2 in, 2 out]
                  }
                }
              }
            }
          }
          event "Shutter": Value Change {
            n2914 = event-data() -> ()  [unwired: 1 in, 5 out]
            n2915 = case shown="False" "Shutter" {
              frame False {
                n2916 = call "shuttercontrol.vi"("command"="close") -> ()  [unwired: 1 in, 1 out]
              }
              frame True {
                n2917 = call "shuttercontrol.vi"("command"="open") -> ()  [unwired: 1 in, 1 out]
              }
            }
          }
          event "ROI": Value Change {
            n2918 = event-data() -> ()  [unwired: 1 in, 5 out]
            n2919 = local read "ROI"() -> (w6031:bool)
            n2920 = case shown="True" w6031 {
              frame False {
              }
              frame True {
                n2921 = stacked-sequence {
                  frame #0 {
                    n2922 = local read "Square pixels"() -> (w6048:bool)
                    n2923 = local read "square matrix"() -> (w6047:bool)
                    n2924 = local read "Vx-max ref"() -> (w6053:dbl)
                    n2925 = local read "Vx-min ref"() -> (w6052:dbl)
                    n2926 = local read "Vy-min ref"() -> (w6049:dbl)
                    n2927 = local read "ypixels ref"() -> (w6051:i32)
                    n2928 = local read "Vy-max ref"() -> (w6050:dbl)
                    n2929 = local read "xpixels ref"() -> (w6054:i32)
                    n2930 = local read "Angle ref"() -> (w6046:dbl)
                    n2931 = local read "Colormap"() -> (w6055:i32)
                    n2932 = call "2pparameters.vi"("command"="get") -> ("params out"=w6058:T12)  [unwired: 1 in]
                    n2933 = Bundle By Name(cluster=w6058, "Xpixels Img"=w6054, "Vx-min Img"=w6052, "VX-max Img"=w6053, "Ypixels Img"=w6051, "Vy-min Img"=w6049, "Vy-max Img"=w6050, "Colormap"=w6055, "square pixels"=w6048, "square matrix"=w6047, "Angle Img"=w6046) -> (w6057:T12)
                    n2934 = call "2pparameters.vi"("Params in"=w6057, "command"="set") -> ()  [unwired: 1 out]
                    n2935 = local read "Vx-max draw"() -> (w6038:dbl)
                    n2936 = local read "Angle drawing"() -> (w6045:dbl)
                    n2937 = local read "Vx-min draw"() -> (w6039:dbl)
                    n2938 = local read "Vy-min draw"() -> (w6042:dbl)
                    n2939 = local read "ypixels draw"() -> (w6040:dbl)
                    n2940 = local read "Vy-max draw"() -> (w6041:dbl)
                    n2941 = local read "Square pixels"() -> (w6043:bool)
                    n2942 = local read "square matrix"() -> (w6044:bool)
                    n2943 = local read "xpixels draw"() -> (w6037:dbl)
                    n2944 = local read "Colormap"() -> (w6036:i32)
                    n2945 = call "2pparameters.vi"("command"="get") -> ("params out"=w6033:T12)  [unwired: 1 in]
                    n2946 = Bundle By Name(cluster=w6033, "Xpixels"=w6037, "Vxminref"=w6039, "Vxmaxref"=w6038, "Ypixels"=w6040, "Vyminref"=w6042, "Vymaxref"=w6041, "Colormap"=w6036, "square pixels"=w6043, "square matrix"=w6044, "Angle draw"=w6045) -> (w6034:T12)
                    n2947 = call "2pparameters.vi"("Params in"=w6034, "command"="set") -> ()  [unwired: 1 out]
                  }
                  frame #1 {
                    n2948 = Current VI's Path() -> (path=w6069:path)
                    n2949 = Strip Path(path=w6069) -> (stripped path=w6070:path)  [unwired: 1 out]
                    n2950 = Build Path(base path=w6070, name or relative path="subVIs\\Image\\SetROI_v3.vi") -> (appended path=w6068:path)
                    n2951 = call <vilib>:"Set Busy.vi"() -> ("error out"=w6066:errorcluster)  [unwired: 10 in, 1 out]
                    n2952 = Open VI Reference(type specifier VI Refnum (for type only)=refnum<vi> refnum, vi path=w6068, error in (no error)=w6066) -> (vi reference=w6064:refnum<vi>, error out=w6062:errorcluster)  [unwired: 3 in]
                    n2953 = call-by-ref "?"(reference=w6064, error in=w6062) -> (reference out=w6063:refnum<vi>, error out=w6061:errorcluster)  [unwired: 1 in]
                    n2954 = Close Reference(reference=w6063, error in (no error)=w6061) -> (error out=w6065:errorcluster)
                    n2955 = call <vilib>:"Unset Busy.vi"("error in (no error)"=w6065) -> ()  [unwired: 10 in, 1 out]
                    n2956 = local write "status"(w6065) -> ()
                  }
                  frame #2 {
                    n2957 = call "2pparameters.vi"("command"="get") -> ("params out"=w6095:T12)  [unwired: 1 in]
                    n2958 = Unbundle By Name(w6095) -> ("Xpixels Img"=w6094:i32, "Vx-min Img"=w6093:dbl, "VX-max Img"=w6092:dbl, "Ypixels Img"=w6091:i32, "Vy-min Img"=w6090:dbl, "Vy-max Img"=w6089:dbl, "Colormap"=w6088:u16, "square pixels"=w6087:bool, "square matrix"=w6086:bool, "Angle Img"=w6085:dbl, "Drawing Mode"=w6084:u16)
                    n2959 = local write "xpixels ref"(w6094) -> ()
                    n2960 = local write "Vx-min ref"(w6093) -> ()
                    n2961 = local write "Vx-max ref"(w6092) -> ()
                    n2962 = local write "ypixels ref"(w6091) -> ()
                    n2963 = local write "Vy-min ref"(w6090) -> ()
                    n2964 = local write "Vy-max ref"(w6089) -> ()
                    n2965 = local write "Colormap"(w6088) -> ()
                    n2966 = local write "Square pixels"(w6087) -> ()
                    n2967 = local write "square matrix"(w6086) -> ()
                    n2968 = local write "Angle ref"(w6085) -> ()
                    n2969 = local write "ROI Type"(w6084) -> ()
                    n2970 = call "2pparameters.vi"("command"="get") -> ("params out"=w6078:T12)  [unwired: 1 in]
                    n2971 = Unbundle By Name(w6078) -> ("Xpixels"=w6072:i32, "Vxminref"=w6076:dbl, "Vxmaxref"=w6075:dbl, "Ypixels"=w6071:i32, "Vyminref"=w6074:dbl, "Vymaxref"=w6073:dbl, "Colormap"=w6079:u16, "square pixels"=w6080:bool, "square matrix"=w6081:bool, "Angle draw"=w6082:dbl, "Drawing Mode"=w6083:u16)
                    n2972 = local write "Vy-max draw"(w6073) -> ()
                    n2973 = local write "Angle drawing"(w6082) -> ()
                    n2974 = local write "Colormap"(w6079) -> ()
                    n2975 = local write "Square pixels"(w6080) -> ()
                    n2976 = local write "square matrix"(w6081) -> ()
                    n2977 = local write "ROI Type"(w6083) -> ()
                    n2978 = local write "xpixels draw"(w6072) -> ()
                    n2979 = local write "ypixels draw"(w6071) -> ()
                    n2980 = local write "Vx-min draw"(w6076) -> ()
                    n2981 = local write "Vx-max draw"(w6075) -> ()
                    n2982 = local write "Vy-min draw"(w6074) -> ()
                  }
                  frame #3 {
                    n2983 = property on="ROI" class="Bool (strict)"("Val(Sgnl)"=FALSE ("x/y scan")) -> ()  [unwired: 2 in, 2 out]
                  }
                }
              }
            }
          }
          event "Xdattype": Value Change {
            n2984 = event-data() -> ()  [unwired: 1 in, 1 out]
            n2985 = case shown="True" "Xdattype" {
              frame False {
              }
              frame True {
                n2986 = stacked-sequence {
                  frame #0 {
                    n2987 = Current VI's Path() -> (path=w6108:path)
                    n2988 = Strip Path(path=w6108) -> (stripped path=w6109:path)  [unwired: 1 out]
                    n2989 = Build Path(base path=w6109, name or relative path="subVIs\\Misc\\Changedataconfig.vi") -> (appended path=w6107:path)
                    n2990 = call <vilib>:"Set Busy.vi"() -> ("error out"=w6105:errorcluster)  [unwired: 10 in, 1 out]
                    n2991 = Open VI Reference(type specifier VI Refnum (for type only)=refnum<vi> refnum, vi path=w6107, error in (no error)=w6105) -> (vi reference=w6100:refnum<vi>, error out=w6102:errorcluster)  [unwired: 3 in]
                    n2992 = call-by-ref "?"(reference=w6100, error in=w6102) -> (reference out=w6104:refnum<vi>, error out=w6103:errorcluster)  [unwired: 12 in]
                    n2993 = Close Reference(reference=w6104, error in (no error)=w6103) -> (error out=w6099:errorcluster)
                    "status" <- w6099
                    n2994 = call <vilib>:"Unset Busy.vi"("error in (no error)"=w6099) -> ()  [unwired: 10 in, 1 out]
                  }
                  frame #1 {
                    n2995 = property on="Xdattype" class="Bool (strict)"("Val(Sgnl)"=FALSE ("x/y scan")) -> ()  [unwired: 2 in, 2 out]
                  }
                }
              }
            }
          }
          event "XautoOD": Value Change {
            n2996 = event-data() -> ()  [unwired: 1 in, 1 out]
            n2997 = case shown="True" "XautoOD" {
              frame False {
              }
              frame True {
                n2998 = stacked-sequence {
                  frame #0 {
                    n2999 = Current VI's Path() -> (path=w6121:path)
                    n3000 = Strip Path(path=w6121) -> (stripped path=w6122:path)  [unwired: 1 out]
                    n3001 = Build Path(base path=w6122, name or relative path="subVIs\\Misc\\ChangeautoODs.vi") -> (appended path=w6120:path)
                    n3002 = call <vilib>:"Set Busy.vi"() -> ("error out"=w6118:errorcluster)  [unwired: 10 in, 1 out]
                    n3003 = Open VI Reference(type specifier VI Refnum (for type only)=refnum<vi> refnum, vi path=w6120, error in (no error)=w6118) -> (vi reference=w6113:refnum<vi>, error out=w6115:errorcluster)  [unwired: 3 in]
                    n3004 = call-by-ref "?"(reference=w6113, error in=w6115) -> (reference out=w6117:refnum<vi>, error out=w6116:errorcluster)  [unwired: 12 in]
                    n3005 = Close Reference(reference=w6117, error in (no error)=w6116) -> (error out=w6112:errorcluster)
                    "status 2" <- w6112
                    n3006 = call <vilib>:"Unset Busy.vi"("error in (no error)"=w6112) -> ()  [unwired: 10 in, 1 out]
                  }
                  frame #1 {
                    n3007 = property on="XautoOD" class="Bool (strict)"("Val(Sgnl)"=FALSE ("x/y scan")) -> ()  [unwired: 2 in, 2 out]
                  }
                }
              }
            }
          }
          event "SetMan": Value Change {
            n3008 = event-data() -> ()  [unwired: 1 in, 1 out]
            n3009 = case shown="True" "SetMan" {
              frame False {
              }
              frame True {
                n3010 = stacked-sequence {
                  frame #0 {
                    w6125 = u16 0 items=["Rectangle", "Circle", "Freeform Boundary", "Freeform Interior"] ("ROI Type")
                    n3011 = local write "ROI Type"(w6125) -> ()
                    n3012 = local read "Square pixels"() -> (w6131:bool)
                    n3013 = case shown="True" w6131 {
                      frame False {
                        n3014 = local read "square matrix"() -> (w6132:bool)
                        n3015 = case shown="False" w6132 {
                          frame False {
                            "ypixels ref" <- "ypixels"
                            "xpixels ref" <- "xpixels"
                          }
                          frame True {
                            n3016 = local read "xpixels"() -> (w6137:i32)
                            n3017 = local read "ypixels"() -> (w6136:i32)
                            n3018 = Max & Min(x=w6137, y=w6136) -> (max(x,y)=w6135:i32)  [unwired: 1 out]
                            n3019 = local write "xpixels ref"(w6135) -> ()
                            n3020 = local write "ypixels ref"(w6135) -> ()
                          }
                        }
                      }
                      frame True {
                        n3021 = local read "square matrix"() -> (w6138:bool)
                        n3022 = case shown="False" w6138 {
                          frame False {
                            n3023 = local read "Vxmax"() -> (w6152:dbl)
                            n3024 = local read "Vx-min"() -> (w6151:dbl)
                            n3025 = local read "Vy-max"() -> (w6147:dbl)
                            n3026 = local read "Vy-min"() -> (w6148:dbl)
                            n3027 = Subtract(x=w6147, y=w6148) -> (x-y=w6149:dbl)
                            n3028 = Subtract(x=w6152, y=w6151) -> (x-y=w6150:dbl)
                            n3029 = Absolute Value(x=w6149) -> (abs(x)=w6140:dbl)
                            n3030 = Absolute Value(x=w6150) -> (abs(x)=w6141:dbl)
                            n3031 = Divide(x=w6141, y=w6140) -> (x/y=w6146:dbl)
                            n3032 = Greater Or Equal?(x=w6141, y=w6140) -> (x >= y?=w6139:bool)
                            n3033 = local read "xpixels"() -> (w6145:i32)
                            n3034 = local read "ypixels"() -> (w6142:i32)
                            n3035 = case shown="False" w6139 {
                              tunnel: w6146 -> [w6157 w6160]
                              tunnel: w6145 -> [w6154 _]
                              tunnel: [w6154 w6159] -> w6144
                              tunnel: [w6153 w6158] -> w6143
                              tunnel: w6142 -> [_ w6158]
                              frame False {
                                n3036 = To Double Precision Float(number=w6154) -> (double precision float=w6156:dbl)
                                n3037 = Divide(x=w6156, y=w6157) -> (x/y=w6155:dbl)
                                n3038 = To Long Integer(number=w6155) -> (32bit integer=w6153:i32)
                              }
                              frame True {
                                n3039 = To Double Precision Float(number=w6158) -> (double precision float=w6162:dbl)
                                n3040 = Multiply(x=w6162, y=w6160) -> (x*y=w6161:dbl)
                                n3041 = To Long Integer(number=w6161) -> (32bit integer=w6159:i32)
                              }
                            }
                            n3042 = local write "ypixels ref"(w6143) -> ()
                            n3043 = local write "xpixels ref"(w6144) -> ()
                          }
                          frame True {
                          }
                        }
                      }
                    }
                    "Vx-max ref" <- "Vxmax"
                    "Vx-min ref" <- "Vx-min"
                    "Vy-max ref" <- "Vy-max"
                    "Vy-min ref" <- "Vy-min"
                    "Angle ref" <- "Angle"
                  }
                  frame #1 {
                    n3044 = property on="SetMan" class="Bool (strict)"("Val(Sgnl)"=FALSE ("Value (Signaling)")) -> ()  [unwired: 2 in, 2 out]
                  }
                }
              }
            }
          }
          event "SetMan 2": Value Change {
            n3045 = event-data() -> ()  [unwired: 1 in, 1 out]
            n3046 = case shown="True" "SetMan 2" {
              frame False {
              }
              frame True {
                n3047 = stacked-sequence {
                  frame #0 {
                    n3048 = local write "Vx-ref"("Vx") -> ()
                    n3049 = local write "Vy-ref"("Vy") -> ()
                  }
                  frame #1 {
                    n3050 = property on="SetMan 2" class="Bool (strict)"("Val(Sgnl)"=FALSE ("Value (Signaling)")) -> ()  [unwired: 2 in, 2 out]
                  }
                }
              }
            }
          }
          event "Reset Coords": Value Change {
            n3051 = event-data() -> ("NewVal"=w6168:bool)  [unwired: 1 in, 5 out]
            n3052 = case shown="True" w6168 {
              frame False {
              }
              frame True {
                n3053 = stacked-sequence {
                  frame #0 {
                    n3054 = local write "xpixels"(256 ("xpixels")) -> ()
                    n3055 = local write "ypixels"(256 ("ypixels")) -> ()
                    n3056 = local write "Vxmax"(9.0 ("Vx-max")) -> ()
                    n3057 = local write "Vx-min"(-9.0 ("Vx-min")) -> ()
                    n3058 = local write "Vy-max"(9.0 ("Vy-max")) -> ()
                    n3059 = local write "Vy-min"(-9.0 ("Vy-min")) -> ()
                    n3060 = local write "Angle"(0.0 ("Angle")) -> ()
                  }
                  frame #1 {
                    n3061 = property on="Reset Coords" class="Bool (strict)"("Value"=FALSE ("TROI")) -> ()  [unwired: 2 in, 2 out]
                  }
                }
              }
            }
          }
          event "TROI": Value Change {
            n3062 = event-data() -> ()  [unwired: 1 in, 1 out]
            n3063 = case shown="True" "TROI" {
              frame False {
              }
              frame True {
                n3064 = stacked-sequence {
                  frame #0 {
                    n3065 = local read "Vy-min ref"() -> (w6182:dbl)
                    n3066 = local read "Vy-max ref"() -> (w6181:dbl)
                    n3067 = local read "Vx-max ref"() -> (w6179:dbl)
                    n3068 = local read "Vx-min ref"() -> (w6180:dbl)
                    n3069 = local read "ypixels ref"() -> (w6184:i32)
                    n3070 = local read "xpixels ref"() -> (w6183:i32)
                    n3071 = local read "Angle ref"() -> (w6178:dbl)
                    n3072 = local write "Angle"(w6178) -> ()
                    n3073 = local write "xpixels"(w6183) -> ()
                    n3074 = local write "Vy-min"(w6182) -> ()
                    n3075 = local write "Vy-max"(w6181) -> ()
                    n3076 = local write "Vx-min"(w6180) -> ()
                    n3077 = local write "ypixels"(w6184) -> ()
                    n3078 = local write "Vxmax"(w6179) -> ()
                  }
                  frame #1 {
                    n3079 = property on="TROI" class="Bool (strict)"("Value"=FALSE ("TROI")) -> ()  [unwired: 2 in, 2 out]
                  }
                }
              }
            }
          }
          event "TROI 2": Value Change {
            n3080 = event-data() -> ()  [unwired: 1 in, 1 out]
            n3081 = case shown="True" "TROI 2" {
              frame False {
              }
              frame True {
                n3082 = stacked-sequence {
                  frame #0 {
                    n3083 = local read "Vx-ref"() -> (w6187:dbl)
                    n3084 = local read "Vy-ref"() -> (w6188:dbl)
                    n3085 = local write "Vx"(w6187) -> ()
                    n3086 = local write "Vy"(w6188) -> ()
                  }
                  frame #1 {
                    n3087 = property on="TROI 2" class="Bool (strict)"("Value"=FALSE ("TROI")) -> ()  [unwired: 2 in, 2 out]
                  }
                }
              }
            }
          }
          event "Square pixels": Value Change {
            n3088 = event-data() -> ()  [unwired: 1 in, 1 out]
            n3089 = case shown="True" "Square pixels" {
              frame False {
              }
              frame True {
                n3090 = property on="square matrix" class="Bool (strict)"("Value"=FALSE ("square matrix")) -> ()  [unwired: 2 in, 2 out]
                n3091 = property on="Square pixels" class="Bool (strict)"("Value"=TRUE ("square matrix")) -> ()  [unwired: 2 in, 2 out]
              }
            }
          }
          event "square matrix": Value Change {
            n3092 = event-data() -> ()  [unwired: 1 in, 1 out]
            n3093 = case shown="True" "square matrix" {
              frame False {
              }
              frame True {
